vi "Тест_буфера_не_правильно.vi"() -> ()   [LabVIEW 2017]
panel:
  out "Кол-во строк массив":i32
  out "second subarray":i32[](array[numeric])
  out "first subarray":i32[](array[numeric])
  out "size(s) 3":i32[](array[numeric])
  out "size(s) 2":i32[](array[numeric])
  out "2-х массив на выходе":dbl[][](array[numeric])
  in  "Размер окна":i32=4
  out "size(s)":i32[](array[numeric])
  out "Выход последовательного массива":dbl[](array[numeric])
  in  "Последовательный массив":i32=16
  out "Array":dbl[][](array[numeric])
  in  "Размер окна буффера":i32
  out "Количество бит":i32
  in  "Количество бит":i32=8
  out "Биты на выходе":dbl[](array[numeric])
  # "3"
  # "15"
  # "7"
  # "3"
  # "7"
  # "15"
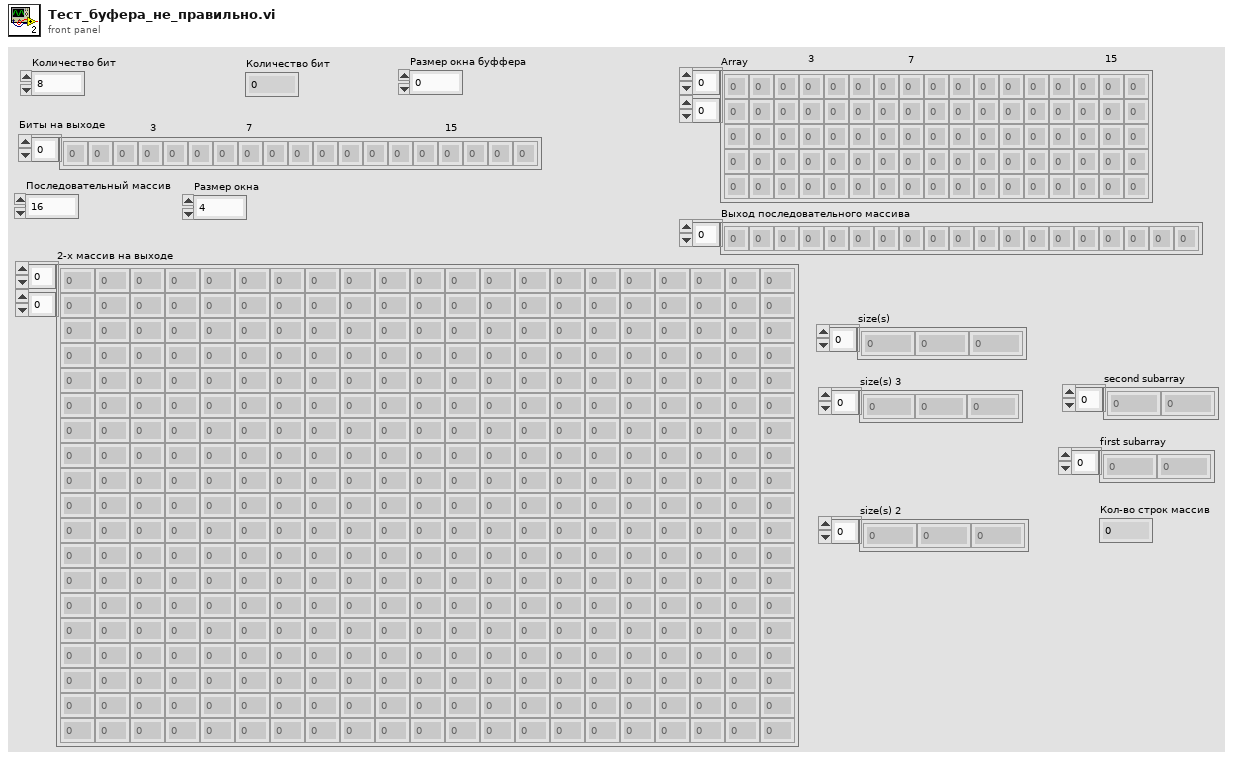
[diagram p1: front panel]
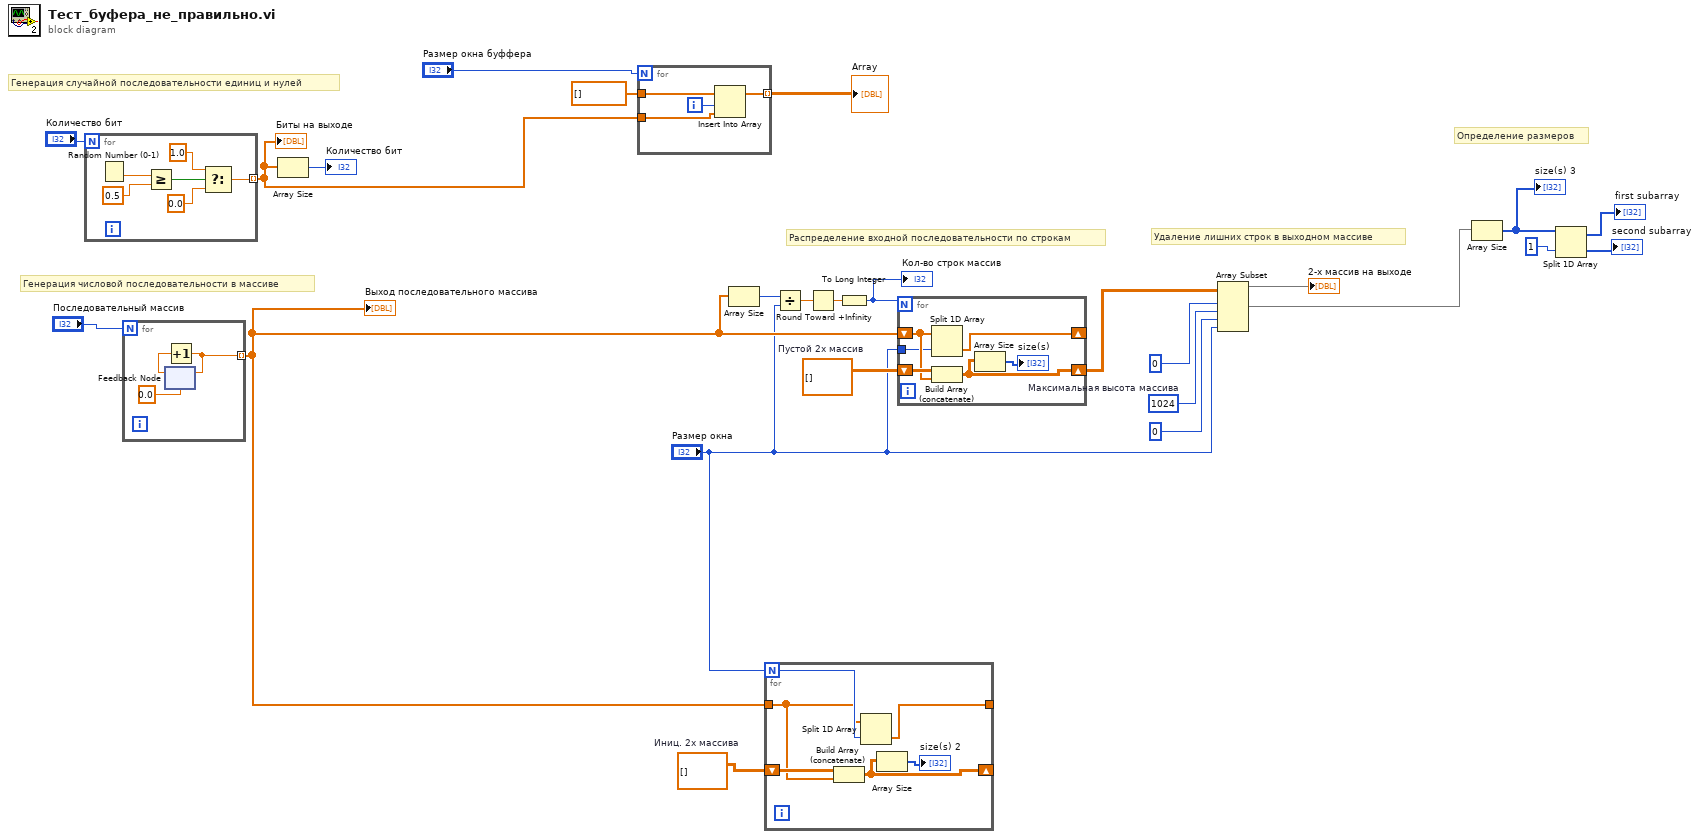
[diagram p0: block diagram]
diagram:
  w12 = dbl[][] []  # Иниц. 2х массива
  w13 = 1024  # Максимальная высота массива
  w17 = dbl[][] []  # Пустой 2х массив
  # "Определение размеров"
  # "Распределение входной последовательности по строкам"
  # "Удаление лишних строк в выходном массиве"
  # "Генерация числовой последовательности в массиве"
  # "Генерация случайной последовательности единиц и нулей"
  n1 = for {
    N: "Количество бит" -> [_]
    tunnel: [w25] -> w19 mode=indexing
    n2 = Random Number (0-1)() -> (number: 0 to 1=w30:dbl)
    n3 = Greater Or Equal?(x=w30, y=0.5) -> (x >= y?=w28:bool)
    n4 = Select(t=1.0, s=w28, f=0.0) -> (s? t:f=w25:dbl)
  }
  "Биты на выходе" <- w19
  n5 = for {
    N: "Последовательный массив" -> [_]
    tunnel: [w31] -> w5 mode=indexing
    n6 = feedback #1(0.0) -> (w33:dbl)
    n7 = Increment(x=w33) -> (x+1=w31:dbl)
    n8 = feedback-in #1(w31) -> ()
  }
  "Выход последовательного массива" <- w5
  n9 = Array Size(array=w19) -> (size(s)=→"Количество бит":i32)
  n10 = for {
    N: "Размер окна буффера" -> [_]
    tunnel: w19 -> [w35]
    tunnel: dbl[] [] -> [w36]
    tunnel: [w37] -> w22 mode=indexing
    i -> [w34]
    n11 = Insert Into Array(array=w36, index=w34, new element=w35) -> (w37:dbl[])
  }
  "Array" <- w22
  n12 = Array Size(array=w5) -> (size(s)=w6:i32)
  n13 = for {
    N: "Размер окна" -> [w40]
    shift-right: [w41] -> _
    shift-left: w12 -> [w39]
    tunnel: w5 -> [w38]
    tunnel: [w42] -> _
    n14 = Build Array (concatenate)(w39, w38) -> (w41:dbl[][])
    n15 = Split 1D Array(array=w38, index=w40) -> (second subarray=w42:dbl[])  [unwired: 1 out]
    n16 = Array Size(array=w41) -> (size(s)=→"size(s) 2":i32[])
  }
  n17 = Divide(x=w6, y="Размер окна") -> (x/y=w4:dbl)
  n18 = Round Toward +Infinity(x=w4) -> (ceil(x): smallest int >= x=w2:dbl)
  n19 = To Long Integer(number=w2) -> (32bit integer=w3:i32)
  "Кол-во строк массив" <- w3
  n20 = for {
    N: w3 -> [_]
    shift-right: [w48] -> w16
    shift-left: w17 -> [w49]
    shift-right: [w46] -> _
    shift-left: w5 -> [w45]
    tunnel: "Размер окна" -> [w44]
    n21 = Split 1D Array(array=w45, index=w44) -> (second subarray=w46:dbl[])  [unwired: 1 out]
    n22 = Build Array (concatenate)(w49, w45) -> (w48:dbl[][])
    n23 = Array Size(array=w48) -> (size(s)=→"size(s)":i32[])
  }
  n24 = Array Subset(array=w16, index (row)=0 ("length"), length (row)=w13, index (col)=0 ("index"), length (col)="Размер окна") -> (w11:dbl[][])
  "2-х массив на выходе" <- w11
  n25 = Array Size(array=w11) -> (size(s)=w10:i32[])
  "size(s) 3" <- w10
  n26 = Split 1D Array(array=w10, index=1) -> (first subarray=→"first subarray":i32[], second subarray=→"second subarray":i32[])
